vi "FPGA PWM test.vi"() -> ()   [LabVIEW 2014]
doc: "This FPGA VI defines the functionality that is needed for the C terminal connector for the myRIO sheepdog robot project. It provides two PWM outputs, two single-line counters (for the Hall effect encoders), and digital IO needed to command the motors. It also determines a measure of the derivative of the encoder counter lines (proportional to wheel speed)."
uses:
  <vilib>/Platform/TimedLoop/XDataNode/timing_clust.ctl
  <vilib>/Platform/TimedLoop/XDataNode/nitl_modes.ctl
  <vilib>/Platform/TimedLoop/XDataNode/wakeup.ctl
  <vilib>/rvi/Emulation/niFpgaSctlEmulationGetInTimedLoop.vi
  <vilib>/rvi/Emulation/niFpgaEmulationReportErrorSimple.vi
  <vilib>/rvi/Emulation/niFpgaGetClockAttributes.vi
  <vilib>/rvi/Emulation/niFpgaCriticalErrorInLSC.vi
  <vilib>/rvi/eio/common/nirviEmuTemplateMethod_errors.vi
  <vilib>/rvi/Emulation/niFpgaProcessEmulError.vi
  <vilib>/Platform/TimedLoop/XDataNode/XDataNode.xnode
  <vilib>/eio/EIONode/EIONode.xnode
  <vilib>/eio/EIOMethodNode/EIOMethodNode.xnode
  <vilib>/Platform/TimedLoop/XDataNode/XDNodeRunTimeDep.lvlib
panel:
  in  "Direction 2":bool
  in  "Direction 1":bool
  in  "Duty Cycle Divisor":i16=30000
  in  "Duty Cycle 2":i16
  in  "Duty Cycle 1":i16
  out "SYS.RDY":bool=TRUE
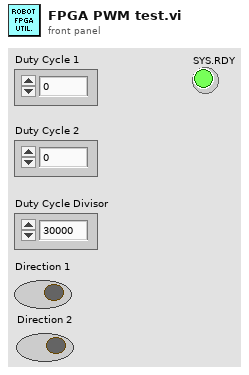
[diagram p1: front panel]
types:
  T1 = typedef "XDNodeRunTimeDep.lvlib/timing_clust.ctl" = cluster{"Expected End [f-1]":u64, "Actual End [f-1]":u64, "Finished Late? [f-1]":bool, "Expected End [i-1]":u64, "Actual End [i-1]":u64, "Finished Late? [i-1]":bool, "Expected Start [i]":u64, "Actual Start [i]":u64, "Expected Start [f]":u64, "Actual Start [f]":u64, "Source Name":string, "Structure Name":string, "Period":i64, "Deadline":i64, "Offset":i64, "Start":i64, "Priority":i32, "Timeout":i32, "Mode":T2, "Wakeup Reason":T3, "Error":errorcluster, "Source Type":string, "Secondary Source Type":string, "Global End Time":u64, "Global Start Time":u64, "Frame Duration":u64, "Iteration Duration":u64, "Assigned CPU":i32, "I/O Scan Engine Mode":u32}
  T2 = typedef "XDNodeRunTimeDep.lvlib/nitl_modes.ctl" = enum32{"No Change", "Process missed periods, maintain original phase", "Discard missed periods, maintain original phase", "Process missed periods, ignore original phase", "Discard missed periods, ignore original phase"}
  T3 = typedef "XDNodeRunTimeDep.lvlib/wakeup.ctl" = enum32{"Normal", "Aborted", "Asynchronous wakeup", "Timing source error", "Timed loop error", "Timeout"}
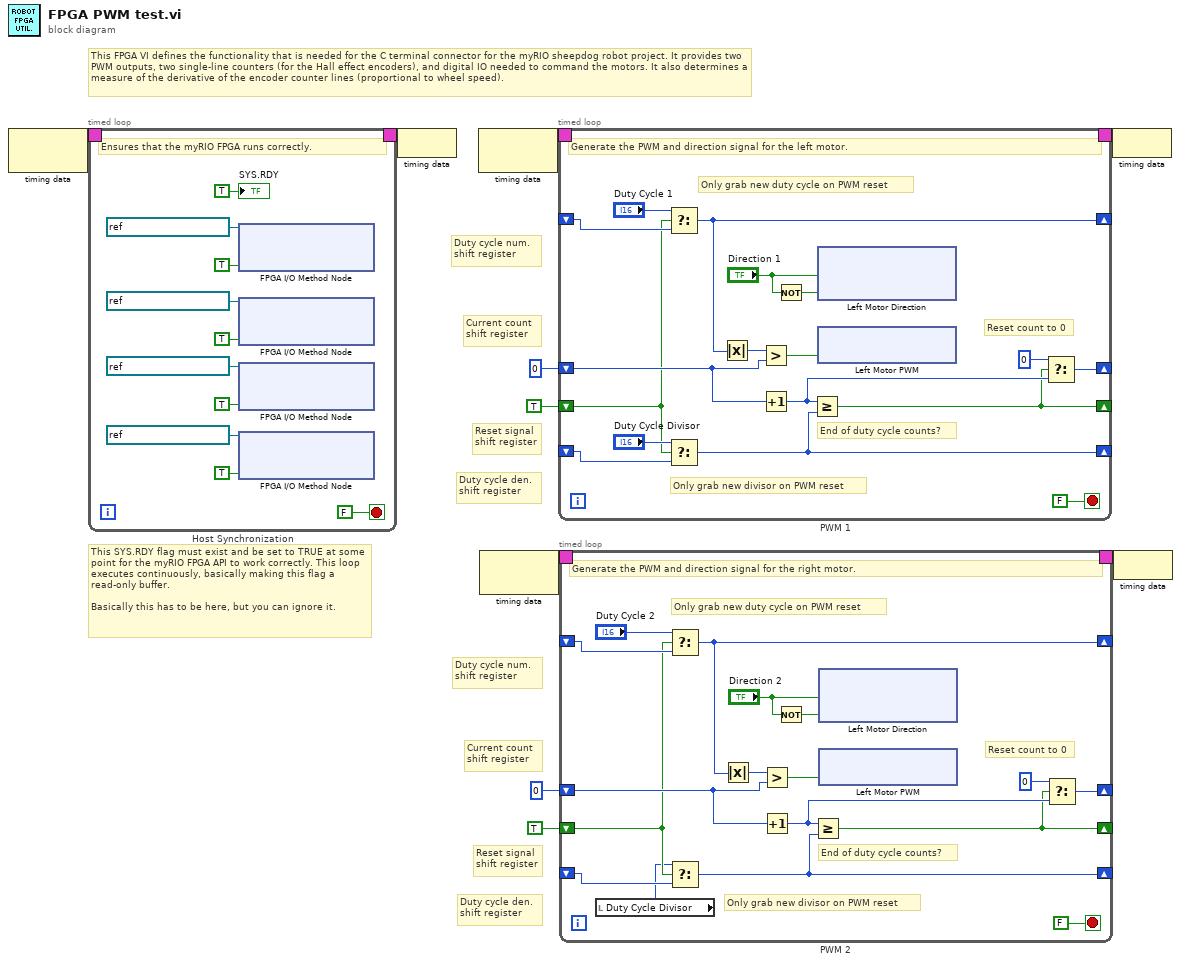
[diagram p0: block diagram]
diagram:
  # "This SYS.RDY flag must exist and be set to TRUE at some point for the myRIO FPGA API to work correctly. This loop executes continuously, basically making this flag a read-only buffer.\n\nBasically this has to be here, but you can ignore it."
  # "Current count\nshift register"
  # "Reset signal\nshift register"
  # "Duty cycle den.\nshift register"
  # "Duty cycle num.\nshift register"
  # "Current count\nshift register"
  # "Reset signal\nshift register"
  # "Duty cycle den.\nshift register"
  # "Duty cycle num.\nshift register"
  # "This FPGA VI defines the functionality that is needed for the C terminal connector for the myRIO sheepdog robot project. It provides two PWM outputs, two single-line counters (for the Hall effect encoders), and digital IO needed to command the motors. It also determines a measure of the derivative of the encoder counter lines (proportional to wheel speed)."
  n1 = node-c288() -> (w2:T1)  [unwired: 1 in]
  n2 = timed-loop "Host Synchronization" {
    timing: w2 -> [_]
    timing-out: [_] -> w1
    stop <- FALSE stop-if-true
    # "Ensures that the myRIO FPGA runs correctly."
    n3 = xnode "FPGA I/O Method Node"("FPGA I/O In"=refnum<k21> "ConnectorC/DIO1", "Enable"=TRUE) -> ()  [unwired: 1 out]
    n4 = xnode "FPGA I/O Method Node"("FPGA I/O In"=refnum<k21> "ConnectorC/DIO3", "Enable"=TRUE) -> ()  [unwired: 1 out]
    n5 = xnode "FPGA I/O Method Node"("FPGA I/O In"=refnum<k21> "ConnectorC/DIO5", "Enable"=TRUE) -> ()  [unwired: 1 out]
    n6 = xnode "FPGA I/O Method Node"("FPGA I/O In"=refnum<k21> "ConnectorC/DIO7", "Enable"=TRUE) -> ()  [unwired: 1 out]
    "SYS.RDY" <- TRUE
  }
  n7 = node-c288(w1) -> ()
  n8 = node-c288() -> (w10:T1)  [unwired: 1 in]
  n9 = node-c288() -> (w6:T1)  [unwired: 1 in]
  n10 = timed-loop "PWM 1" {
    timing: w10 -> [_]
    timing-out: [_] -> w9
    shift-right: [w37] -> _
    shift-left: _ -> [w38]
    shift-right: [w31] -> _
    shift-left: i16 0 -> [w34]
    shift-right: [w29] -> _
    shift-left: TRUE -> [w27]
    shift-right: [w26] -> _
    shift-left: _ -> [w25]
    stop <- FALSE stop-if-true
    # "Only grab new divisor on PWM reset"
    # "End of duty cycle counts?"
    # "Reset count to 0"
    # "Only grab new duty cycle on PWM reset"
    # "Generate the PWM and direction signal for the left motor."
    n11 = Select(t="Duty Cycle 1", s=w27, f=w38) -> (s? t:f=w37:i16)
    n12 = Select(t="Duty Cycle Divisor", s=w27, f=w25) -> (s? t:f=w26:i16)
    n13 = Absolute Value(x=w37) -> (abs(x)=w36:i16)
    n14 = Greater?(x=w36, y=w34) -> (0:w35:bool)
    n15 = Increment(x=w34) -> (x+1=w33:i16)
    n16 = Not(x="Direction 1") -> (.not. x?=w24:bool)
    n17 = Greater Or Equal?(x=w33, y=w26) -> (x >= y?=w29:bool)
    n18 = xnode "Left Motor Direction"("ConnectorC/DIO0"="Direction 1", "ConnectorC/DIO1"=w24) -> ()  [unwired: 2 in, 2 out]
    n19 = xnode "Left Motor PWM"("ConnectorC/DIO3"=w35) -> ()  [unwired: 1 in, 1 out]
    n20 = Select(t=i16 0, s=w29, f=w33) -> (s? t:f=w31:i16)
  }
  n21 = timed-loop "PWM 2" {
    timing: w6 -> [_]
    timing-out: [_] -> w5
    shift-right: [w57] -> _
    shift-left: _ -> [w58]
    shift-right: [w51] -> _
    shift-left: i16 0 -> [w54]
    shift-right: [w49] -> _
    shift-left: TRUE -> [w48]
    shift-right: [w47] -> _
    shift-left: _ -> [w46]
    stop <- FALSE stop-if-true
    # "Only grab new divisor on PWM reset"
    # "End of duty cycle counts?"
    # "Reset count to 0"
    # "Only grab new duty cycle on PWM reset"
    # "Generate the PWM and direction signal for the right motor."
    n22 = local read "Duty Cycle Divisor"() -> (w44:i16)
    n23 = Select(t="Duty Cycle 2", s=w48, f=w58) -> (s? t:f=w57:i16)
    n24 = Select(t=w44, s=w48, f=w46) -> (s? t:f=w47:i16)
    n25 = Absolute Value(x=w57) -> (abs(x)=w56:i16)
    n26 = Greater?(x=w56, y=w54) -> (0:w55:bool)
    n27 = Increment(x=w54) -> (x+1=w53:i16)
    n28 = Not(x="Direction 2") -> (.not. x?=w43:bool)
    n29 = Greater Or Equal?(x=w53, y=w47) -> (x >= y?=w49:bool)
    n30 = xnode "Left Motor Direction"("ConnectorC/DIO4"="Direction 2", "ConnectorC/DIO5"=w43) -> ()  [unwired: 2 in, 2 out]
    n31 = xnode "Left Motor PWM"("ConnectorC/DIO7"=w55) -> ()  [unwired: 1 in, 1 out]
    n32 = Select(t=i16 0, s=w49, f=w53) -> (s? t:f=w51:i16)
  }
  n33 = node-c288(w9) -> ()
  n34 = node-c288(w5) -> ()
